vi "parse user data message.vi"(11 "message":refnum<class "communicator message.lvclass">) -> (1 "invalid?":bool, 3 "data":refnum<class "communicator message.lvclass">)   [LabVIEW 2015, in "queue manager.lvclass"]
uses:
  queue manager.lvclass
  message/communicator message.lvclass
  message/communicator message.lvclass/communicator message.ctl
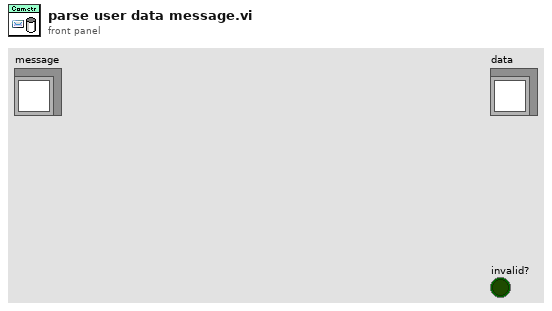
[diagram p1: front panel]
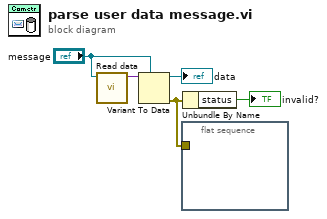
[diagram p0: block diagram]
diagram:
  n1 = call "Read data.vi"("communicator message in"="message") -> ("data"=w5:variant)  [unwired: 10 in]
  n2 = Variant To Data(type="message", Variant=w5) -> (data=→"data":refnum<class "communicator message.lvclass">, error out=w4:errorcluster)  [unwired: 1 in]
  n3 = flat-sequence {
    tunnel: w4 -> [_]
    frame #0 {
    }
  }
  n4 = Unbundle By Name(w4) -> ("status"=→"invalid?":bool)
